vi "PH_gentec_Powermeter.set Trigger Level.vi"(0 "i ref in":refnum<vi>, 2 "VISA resource in":refnum<visa-resource-name>, 4 "Device error in":errorcluster, 5 "error in":errorcluster) -> (13 "Settings changed":bool, 14 "i ref out":refnum<vi>, 15 "Timeout":bool, 16 "VISA resource out":refnum<visa-resource-name>, 17 "Error Message":string, 18 "Device error out":errorcluster, 19 "error out":errorcluster)   [LabVIEW 2014, in "PH_gentec_Powermeter.lvlib"]
doc: "This VI sets the trigger level of the powermeter. Then the value verified by the powermeter is passed to own attributes and the GUI element."
uses:
  PH_gentec_Powermeter.lvlib
  non_GPL/instr.lib/gentec-SOLO-PE/gentec-SOLO-PE - Driver.lvlib
  PH_Powermeter_BaseClass/PH_Powermeter_BaseClass.lvlib
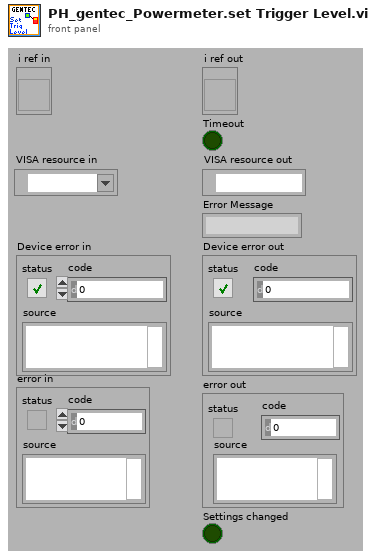
[diagram p1: front panel]
types:
  T1 = typedef "PH_Powermeter_BaseClass.lvlib/PH_Powermeter_BaseClass.i attribute.ctl" = cluster{"GUI References":T2, "Connection":T3, "Head Attributes":T5, "VISA resource":refnum<visa-resource-name>, "Energy":T6, "Service ID Energy":i32, "Wanted Settings":T7, "Current Settings":T7}
  T2 = typedef "PH_Powermeter_BaseClass.lvlib/PH_Powermeter_BaseClass.GUI Refs.ctl" = cluster{"Head Attributes":refnum<vi>, "Energy":refnum<vi>, "Connection":refnum<vi>, "VISA Resource":refnum<vi>, "Energy evolution":refnum<vi>, "Scaling Factor":refnum<vi>, "Range":refnum<vi>, "Wavelength":refnum<vi>, "Trigger Level":refnum<vi>, "Wanted Settings":refnum<vi>, "Current Settings":refnum<vi>}
  T3 = typedef "PH_Powermeter_BaseClass.lvlib/PH_Powermeter_BaseClass.Connection.ctl" = cluster{"failed checks":i8, "Timeout":bool, "Data read":string, "Failure":bool, "Error":bool, "State":T4}
  T4 = typedef "PH_Powermeter_BaseClass.lvlib/PH_Powermeter_BaseClass.State.ctl" = enum32{"off", "operating", "opened", "checked", "connected", "Sets to change", "running"}
  T5 = typedef "PH_Powermeter_BaseClass.lvlib/PH_Powermeter_BaseClass.Head Attributes.ctl" = cluster{"Instrument Type":string, "Head Version":string, "Head Name":string, "Serial Number":string, "Firmware":string, "Sensor Type":string, "MinimumRange":u32, "Maximum Range":u32, "Min Wavelength":i32, "Max Wavelength":i32}
  T6 = typedef "PH_Powermeter_BaseClass.lvlib/PH_Powermeter_BaseClass.Energy.ctl" = cluster{"current Value":dbl, "unscaled":dbl, "Scaling Factor":dbl}
  T7 = typedef "PH_Powermeter_BaseClass.lvlib/PH_gentec_BaseClass.Head Settings.ctl" = cluster{"Trigger Level":dbl, "Wavelength":u32, "Range":u32}
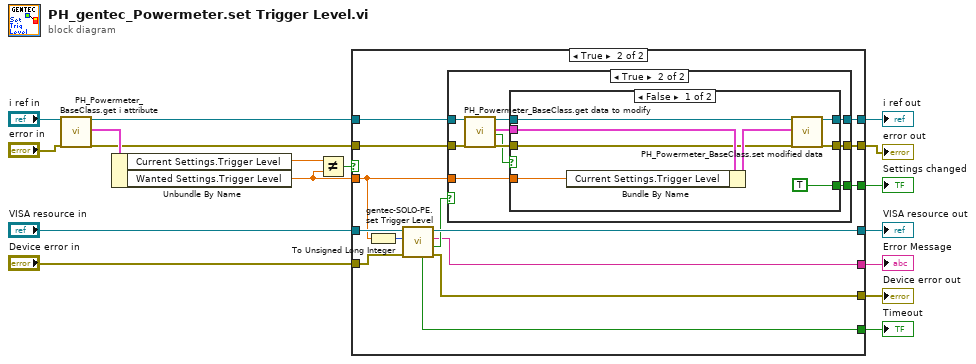
[diagram p0: block diagram]
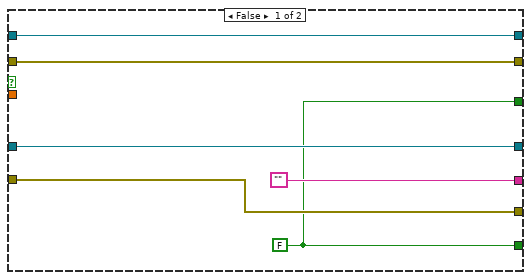
[diagram p2: hidden frame]
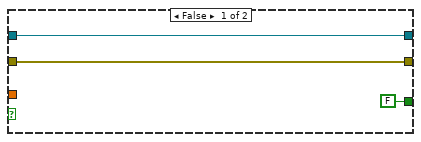
[diagram p3: hidden frame]
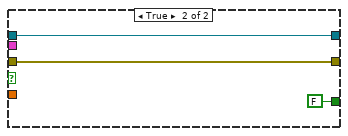
[diagram p4: hidden frame]
diagram:
  n1 = call "PH_Powermeter_BaseClass.get i attribute.vi"("i ref in"="i ref in", "error in (no error)"="error in") -> ("i ref out"=w9:refnum<vi>, "i attribute"=w13:T1, "error out"=w8:errorcluster)  [unwired: 15 in]
  n2 = Unbundle By Name(w13) -> ("Current Settings.Trigger Level"=w12:dbl, "Wanted Settings.Trigger Level"=w11:dbl)
  n3 = Not Equal?(x=w12, y=w11) -> (x != y?=w6:bool)
  n4 = case shown="True" w6 {
    tunnel: [w23 w37] -> w17
    tunnel: [w22 w36] -> w15
    tunnel: w11 -> [_ w29]
    tunnel: "VISA resource in" -> [w21 w34]
    tunnel: w9 -> [w23 w35]
    tunnel: w8 -> [w22 w31]
    tunnel: [w21 w30] -> w7
    tunnel: [w20 w32] -> w5
    tunnel: "Device error in" -> [w20 w33]
    tunnel: ["" w26] -> w2
    tunnel: [w18 w25] -> w3
    tunnel: [w18 w24] -> w1
    frame False {
      w18 = FALSE ("Timeout")
    }
    frame True {
      n5 = To Unsigned Long Integer(number=w29) -> (unsigned 32bit integer=w28:u32)
      n6 = call "gentec-SOLO-PE.set Trigger Level.vi"("error in (no error)"=w33, "Trigger Level (2%)"=w28, "VISA Refnum in"=w34) -> ("error out"=w32:errorcluster, "Acknoledged?"=w27:bool, "Error"=w26:string, "VISA Refnum out"=w30:refnum<visa-resource-name>, "Timeout"=w25:bool)  [unwired: 4 in]
      n7 = case shown="True" w27 {
        tunnel: [w40 w46] -> w37
        tunnel: [w39 w45] -> w36
        tunnel: w35 -> [w40 w44]
        tunnel: w31 -> [w39 w43]
        tunnel: w29 -> [_ w42]
        tunnel: [FALSE w41] -> w24
        frame False {
        }
        frame True {
          n8 = call "PH_Powermeter_BaseClass.get data to modify.vi"("i ref in"=w44, "error in (no error)"=w43) -> ("i ref out"=w50:refnum<vi>, "i attribute"=w49:T1, "timed out"=w47:bool, "error out"=w48:errorcluster)  [unwired: 14 in]
          n9 = case shown="False" w47 {
            tunnel: w48 -> [w55 w60]
            tunnel: w50 -> [w58 w61]
            tunnel: [w53 w61] -> w46
            tunnel: [w52 w60] -> w45
            tunnel: w49 -> [w57 _]
            tunnel: w42 -> [w51 _]
            tunnel: [TRUE FALSE] -> w41
            frame False {
              n10 = Bundle By Name(cluster=w57, "Current Settings.Trigger Level"=w51) -> (w56:T1)
              n11 = call "PH_Powermeter_BaseClass.set modified data.vi"("i ref in"=w58, "i attribute"=w56, "error in (no error)"=w55) -> ("i ref out"=w53:refnum<vi>, "error out"=w52:errorcluster)  [unwired: 15 in]
            }
            frame True {
            }
          }
        }
      }
    }
  }
  "error out" <- w15
  "i ref out" <- w17
  "VISA resource out" <- w7
  "Device error out" <- w5
  "Timeout" <- w3
  "Error Message" <- w2
  "Settings changed" <- w1
